vi "Practica12_ServoEthernet.vi"() -> ()   [LabVIEW 2015]
panel:
  in  "stop":bool
  in  "Dial":u8(knob) scale=0.0..180.0
  # "Servo"
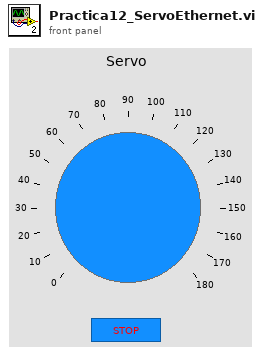
[diagram p1: front panel]
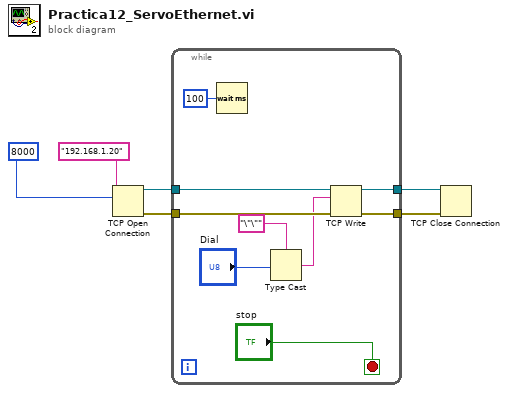
[diagram p0: block diagram]
diagram:
  n1 = TCP Open Connection(address="192.168.1.20", remote port or service name=u16 8000) -> (connection ID=w6:refnum<k5>, error out=w5:errorcluster)  [unwired: 3 in]
  n2 = while {
    tunnel: w6 -> [w15]
    tunnel: w5 -> [w14]
    tunnel: [w12] -> w2
    tunnel: [w11] -> w1
    stop <- "stop" stop-if-true
    n3 = Wait (ms)(milliseconds to wait=u32 100) -> ()  [unwired: 1 out]
    n4 = Type Cast(type="\"\"", x="Dial") -> (*(type *) &x=w9:string)
    n5 = TCP Write(connection ID=w15, data in=w9, error in (no error)=w14) -> (connection ID out=w12:refnum<k5>, error out=w11:errorcluster)  [unwired: 1 in, 1 out]
  }
  n6 = TCP Close Connection(connection ID=w2, error in (no error)=w1) -> ()  [unwired: 1 in, 2 out]
